vi "test Add-Get-Remove Port.vi"(8 "error in":errorcluster, 11 "TestCase in":refnum<class "Scripting.lvclass">) -> (0 "error out":errorcluster, 3 "TestCase out":refnum<class "Scripting.lvclass">)   [LabVIEW 2020, in "Scripting.lvclass"]
uses:
  Scripting.lvclass
  <vilib>/addons/_JKI Toolkits/VI Tester/TestCase.llb/TestCase.lvclass
  Scripting/AIM MIL-STD-1553 Scripting.lvlib
  <vilib>/NI VeriStand/Custom Device API/Custom Device Item Ref.ctl
  <vilib>/NI VeriStand/Custom Device API/Custom Device API.lvlib
  C:/dev/git/niveristand-custom-device-testing-tools/VeriStandScriptingTestCase/VeriStandScriptingTestCase.lvclass
  C:/Program Files (x86)/National Instruments/LabVIEW 2020/vi.lib/addons/_JKI Toolkits/VI Tester/TestCase.llb/TestCase.lvclass
  C:/dev/git/niveristand-aim-milStd1553-custom-device/Source/Custom Device Support/Tests/Unit/Scripting/Scripting.lvclass
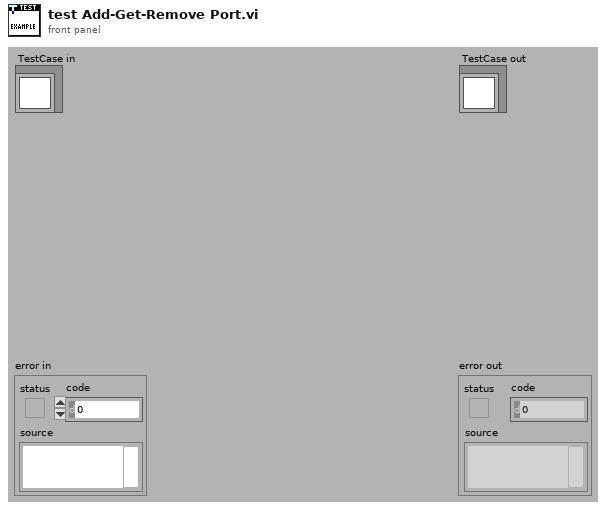
[diagram p1: front panel]
types:
  T1 = typedef "Custom Device API.lvlib/Custom Device Item Ref.ctl" = u64
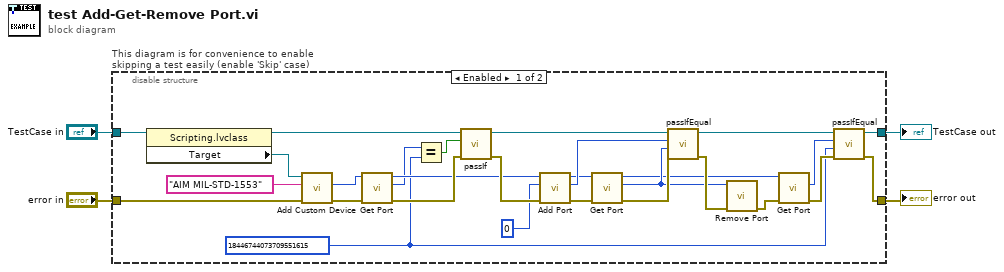
[diagram p0: block diagram]
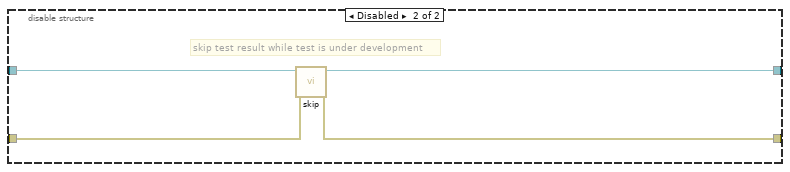
[diagram p2: hidden frame]
diagram:
  n1 = disable-structure "This diagram is for convenience to enable skipping a test easily (enable 'Skip' case)" shown="Enabled" {
    disable-tunnel: "TestCase in" -> [w30 w36]
    disable-tunnel: [w13 w34] -> w1
    disable-tunnel: [w14 w35] -> w3
    disable-tunnel: "error in" -> [w32 w33]
    frame Enabled {
      w6 = T1 18446744073709551615 ("port")
      n2 = property class="Scripting.lvclass"(reference=w30) -> (reference out=w28:refnum<class "Scripting.lvclass">, "Target"=w29:refnum<k24>)  [unwired: 1 in, 1 out]
      n3 = call "Add Custom Device.vi"("error in"=w32, "name"="AIM MIL-STD-1553", "target in"=w29) -> ("error out"=w11:errorcluster, "Ballard MIL-STD 1553 custom device"=w8:T1)  [unwired: 6 in, 1 out]
      n4 = call "Get Port.vi"("error in"=w11, "custom device ref"=w8) -> ("error out"=w10:errorcluster, "port"=w7:T1, "custom device ref out"=w9:T1)  [unwired: 7 in]
      n5 = Equal?(x=w7, y=w6) -> (x = y?=w5:bool)
      n6 = call-dynamic "passIf.vi"("error in (no error)"=w10, "pass"=w5, "TestCase in"=w28) -> ("error out"=w27:errorcluster, "TestCase out"=w26:refnum<class "Scripting.lvclass">)  [unwired: 7 in]
      n7 = call "Add Port.vi"("error in"=w27, "port number"=0, "custom device ref"=w9) -> ("error out"=w22:errorcluster, "port"=w25:T1, "custom device ref out"=w21:T1)  [unwired: 6 in]
      n8 = call "Get Port.vi"("error in"=w22, "custom device ref"=w21) -> ("error out"=w19:errorcluster, "port"=w18:T1, "custom device ref out"=w16:T1)  [unwired: 7 in]
      n9 = call-dynamic "passIfEqual.vi"("error in (no error)"=w19, "y"=w18, "x"=w25, "TestCase in"=w26) -> ("error out"=w23:errorcluster, "TestCase out"=w24:refnum<class "Scripting.lvclass">)  [unwired: 6 in]
      n10 = call "Remove Port.vi"("error in"=w23, "port"=w18) -> ("error out"=w17:errorcluster)  [unwired: 9 in]
      n11 = call "Get Port.vi"("error in"=w17, "custom device ref"=w16) -> ("error out"=w15:errorcluster, "port"=w12:T1)  [unwired: 7 in, 1 out]
      n12 = call-dynamic "passIfEqual.vi"("error in (no error)"=w15, "y"=w6, "x"=w12, "TestCase in"=w24) -> ("error out"=w14:errorcluster, "TestCase out"=w13:refnum<class "Scripting.lvclass">)  [unwired: 6 in]
    }
    frame Disabled {
      # "skip test result while test is under development"
      n13 = call <vilib>:"skip.vi"("error in (no error)"=w33, "TestCase in"=w36) -> ("error out"=w35:errorcluster, "TestCase out"=w34:refnum<class "Scripting.lvclass">)  [unwired: 8 in]
    }
  }
  "error out" <- w3
  "TestCase out" <- w1
